vi "Process.vi"(8 "error in":errorcluster, 11 "Inst UI.Krohn-Hite-7008":refnum<class "Inst UI.Krohn-Hite-7008.lvclass">) -> (0 "error out":errorcluster, 3 "Inst UI.Krohn-Hite-7008 out":refnum<class "Inst UI.Krohn-Hite-7008.lvclass">)   [LabVIEW 2019, in "Inst UI.Krohn-Hite-7008.lvclass"]
doc: "---------------------------------------------------------------\nJKI State Machine Objects™\nhttp://jki.net/state-machine-objects/\nCopyright (C) 2005-2015, JKI <info@jki.net>\nALL RIGHTS RESERVEDJKI State Machine Objects (SMO) 1.0.0.5\nJKI - JKI\nCopyright (c) 2016, JKI"
uses:
  Inst UI.Krohn-Hite-7008.lvclass
  <vilib>/JKI/JKI SMO/SMO/SMO.lvclass
  <vilib>/JKI/JKI SMO/SMO.UI/SMO.UI.lvclass
  <userlib>/LevyLab/Instrument Framework/SMOs/Instrument/Instrument.lvclass
  Inst.Krohn-Hite-7008/Typedefs/Inst.Krohn-Hite-7008.getAll--Cluster.ctl
  Inst.Krohn-Hite-7008/Inst.Krohn-Hite-7008.lvclass
  <userlib>/LevyLab/Instrument Framework/SMOs/Instrument UI/Instrument UI.lvclass
  Inst UI.Krohn-Hite-7008.UI--Cluster.ctl
  <userlib>/LevyLab/Instrument Framework/SMOs/Configuration/Configuration.lvclass
  Inst.Krohn-Hite-7008/Typedefs/Inst.Krohn-Hite-7008.Configuration--Cluster.ctl
  <userlib>/LevyLab/Instrument Framework/SMOs/Instrument/Typedefs/Client Type--Enum.ctl
  <userlib>/LevyLab/Instrument Framework/SMOs/RemoteControl/Typedefs/Message--Cluster.ctl
  <userlib>/LevyLab/Instrument Framework/SMOs/RemoteControl/RemoteControl.lvclass
  09e9697b-516c-49fb-b2dc-692589121b6f.vi
  C:/Program Files (x86)/National Instruments/LabVIEW 2019/user.lib/LevyLab/Instrument Framework/SMOs/Instrument UI/Instrument UI.lvclass
  C:/Program Files (x86)/National Instruments/LabVIEW 2019/vi.lib/JKI/JKI SMO/SMO.UI/SMO.UI.lvclass
  C:/Program Files (x86)/National Instruments/LabVIEW 2019/vi.lib/JKI/JKI SMO/SMO/SMO.lvclass
  Inst.Krohn-Hite-7008/Typedefs/Input Configuration-Enum.ctl
  Inst.Krohn-Hite-7008/Typedefs/Coupling-Enum.ctl
  Inst.Krohn-Hite-7008/Typedefs/Shunt-Enum.ctl
  Inst.Krohn-Hite-7008/Typedefs/Filter-Enum.ctl
  Inst.Krohn-Hite-7008/Typedefs/Gain-Enum.ctl
  Inst.Krohn-Hite-7008/Typedefs/Channel-Enum.ctl
  Inst.Krohn-Hite-7008/Typedefs/SetAll-Cluster.ctl
  Inst.Krohn-Hite-7008/Typedefs/SetAll-Array.ctl
  C:/Program Files (x86)/National Instruments/LabVIEW 2019/user.lib/LevyLab/Instrument Framework/Instrument Types/VSource/Instrument.VSource.lvclass
  C:/Program Files (x86)/National Instruments/LabVIEW 2019/user.lib/LevyLab/Instrument Framework/SMOs/Instrument/Instrument.lvclass
panel:
  out "Serial No":string
  out "Model":string
  in  "Channel Setting":T1
  in  "Parameter 2":string
  out "Numeric":u32
  in  "Update":bool
  in  "Parameter":dbl
  in  "STOP":bool
  # "SMO UI Template"
  # "For instructions on how to use the JKI State Machine Objects, examples and video tutorials, visit:\nhttp://jki.net/state-machine-objects/\n\nJKI State Machine Objects™\nhttp://jki.net/state-machine-objects/\nCopyright (C) 2005-2015, JKI <info@jki.net>\nALL RIGHTS RESERVED"
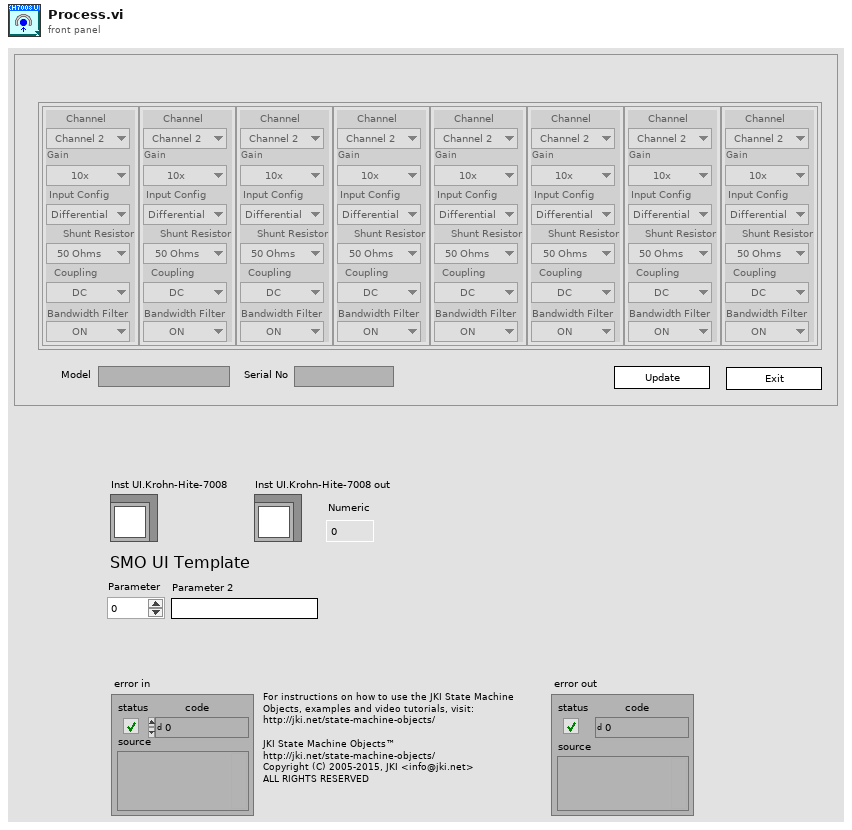
[diagram p1: front panel]
types:
  T1 = typedef "Inst.Krohn-Hite-7008.lvclass/SetAll-Array.ctl" = T2[]
  T2 = typedef "Inst.Krohn-Hite-7008.lvclass/SetAll-Cluster.ctl" = cluster{"Channel":T3, "Gain":T4, "Input Config":T5, "Shunt Resistor":T6, "Coupling":T7, "Bandwidth Filter":T8}
  T3 = typedef "Inst.Krohn-Hite-7008.lvclass/Channel-Enum.ctl" = enum16{"Channel 1", "Channel 2", "Channel 3", "Channel 4", "Channel 5", "Channel 6", "Channel 7", "Channel 8"}
  T4 = typedef "Inst.Krohn-Hite-7008.lvclass/Gain-Enum.ctl" = enum16{"1x", "10x", "100x", "1000x"}
  T5 = typedef "Inst.Krohn-Hite-7008.lvclass/Input Configuration-Enum.ctl" = enum16{"Ground", "SE+ (-gnd)", "SE- (+gnd)", "Differential"}
  T6 = typedef "Inst.Krohn-Hite-7008.lvclass/Shunt-Enum.ctl" = enum16{"Open", "50 Ohms", "500 Ohms", "5k Ohms", "50k Ohms", "10M Ohm"}
  T7 = typedef "Inst.Krohn-Hite-7008.lvclass/Coupling-Enum.ctl" = enum16{"AC", "DC"}
  T8 = typedef "Inst.Krohn-Hite-7008.lvclass/Filter-Enum.ctl" = enum16{"OFF", "ON"}
  T9 = typedef "Inst.Krohn-Hite-7008.lvclass/Inst.Krohn-Hite-7008.Configuration--Cluster.ctl" = cluster{"Visa Ref":refnum<visa-resource-name>, "Serial No":string, "Model":string}
  T10 = enum32{"invalid app kind", "Development System", "Run Time System", "Student Edition", "Embedded LabVIEW", "Evaluation", "Custom"}
  T11 = enum32{"Invalid", "Standard", "Closed", "Hidden", "Minimized", "Maximized"}
  T12 = typedef "Instrument.lvclass/Client Type--Enum.ctl" = enum16{"Remote", "Local"}
  T13 = typedef "Inst.Krohn-Hite-7008.lvclass/Inst.Krohn-Hite-7008.getAll--Cluster.ctl" = cluster{"Levy 1":dbl, "Logger SMO":dbl, "SMO Boolean":bool, "SMO String":string, "Channel Setting":T1}
  T14 = typedef "Inst UI.Krohn-Hite-7008.lvclass/Inst UI.Krohn-Hite-7008.UI--Cluster.ctl" = cluster{"Parameter":dbl, "Parameter 2":string}
  T15 = typedef "RemoteControl.lvclass/Message--Cluster.ctl" = cluster{"Command":string, "Data":variant, "ID":string}
  T16 = cluster{"Core":cluster{"Current VI Reference":refnum<vi>, "Close Panel on Exit?":bool, "Last Error":cluster{"error":errorcluster, "previous state":string, "remaining states":string}, "Shutdown?":bool}, "Instrument UI":refnum<class "Inst UI.Krohn-Hite-7008.lvclass">, "Instrument":refnum<class "Inst.Krohn-Hite-7008.lvclass">, "Configuration":refnum<class "Configuration.lvclass">, "Config Cluster":T9, "getAll":T13, "UI Cluster":T14, "Message":T15}
  T17 = cluster{"Current VI Reference":refnum<vi>, "Close Panel on Exit?":bool, "Last Error":cluster{"error":errorcluster, "previous state":string, "remaining states":string}, "Shutdown?":bool}
  T18 = typedef "SMO.lvclass/Protected Events.ctl" = cluster{"StopProcesses":refnum<user-event>, "AbortProcesses":refnum<user-event>, "Config Changed":refnum<user-event>, "Dependency":refnum<user-event>}
  T19 = typedef "Instrument.lvclass/PublicEvents--Cluster.ctl" = cluster{"MessageFromProcess":refnum<user-event>}
  T20 = typedef "Inst.Krohn-Hite-7008.lvclass/PublicEvents--Cluster.ctl" = cluster{"MessageFromProcess":refnum<user-event>}
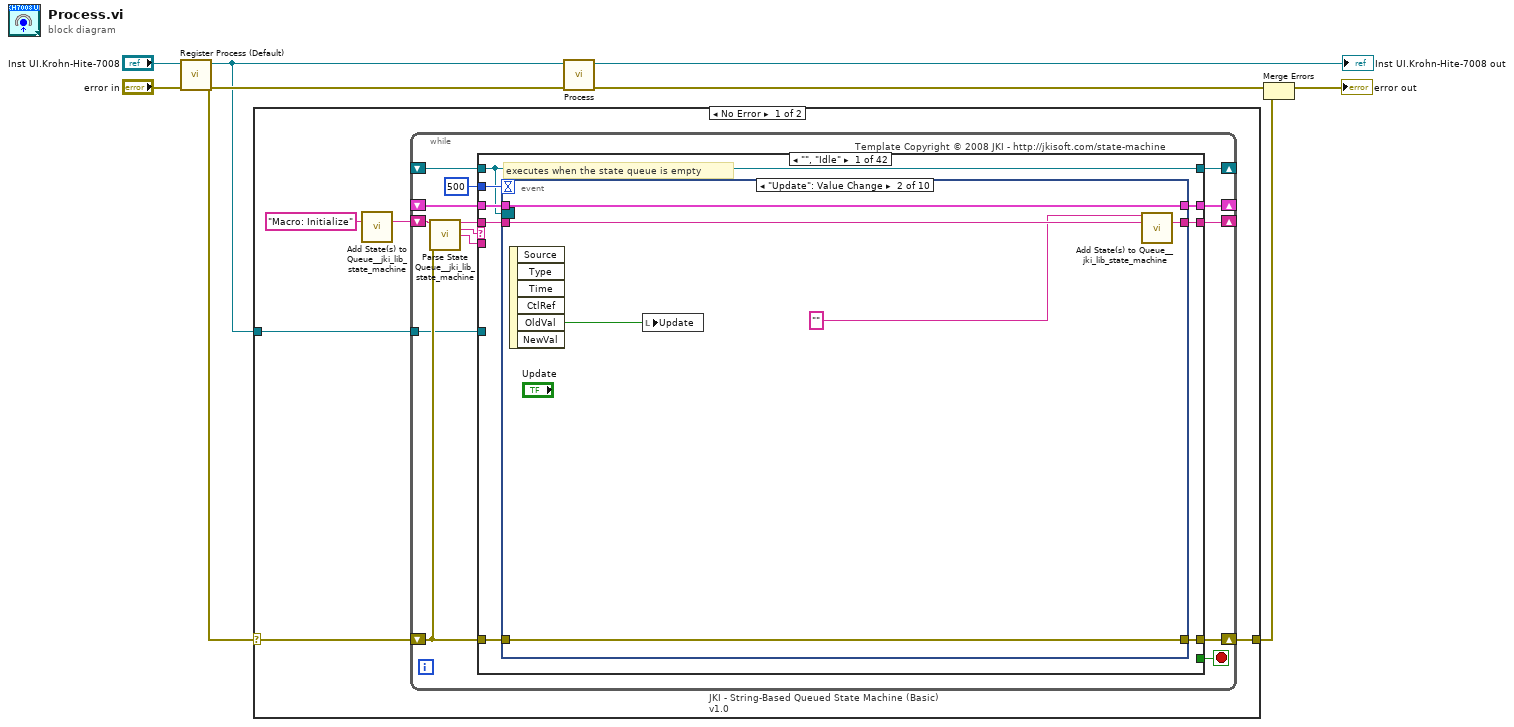
[diagram p0: block diagram]
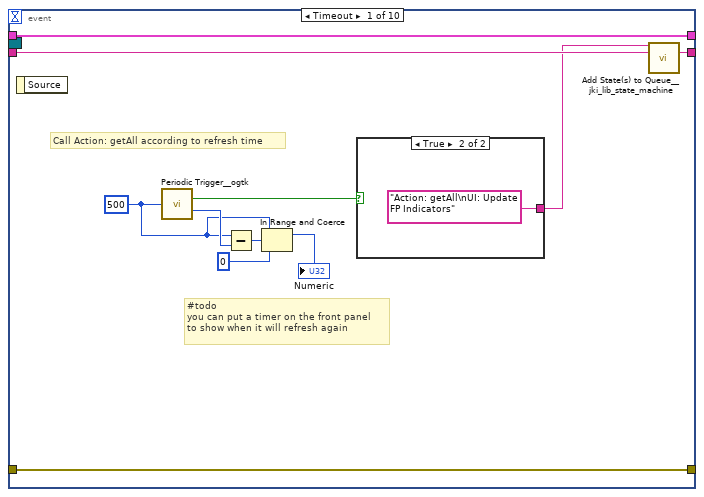
[diagram p2: hidden frame]
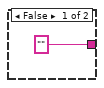
[diagram p3: hidden frame]
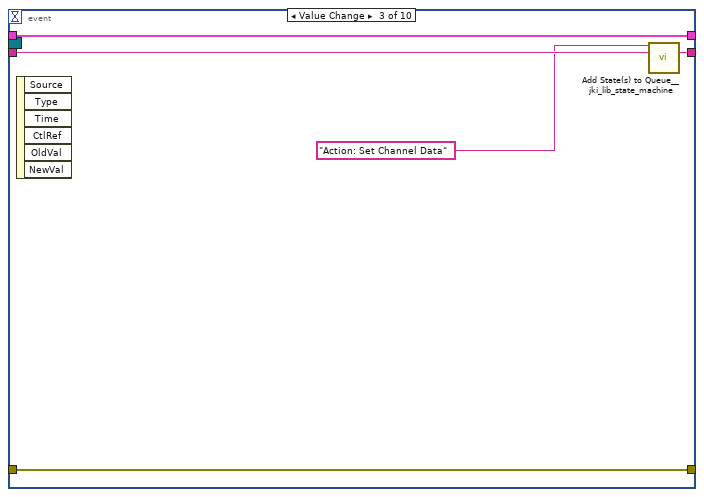
[diagram p4: hidden frame]
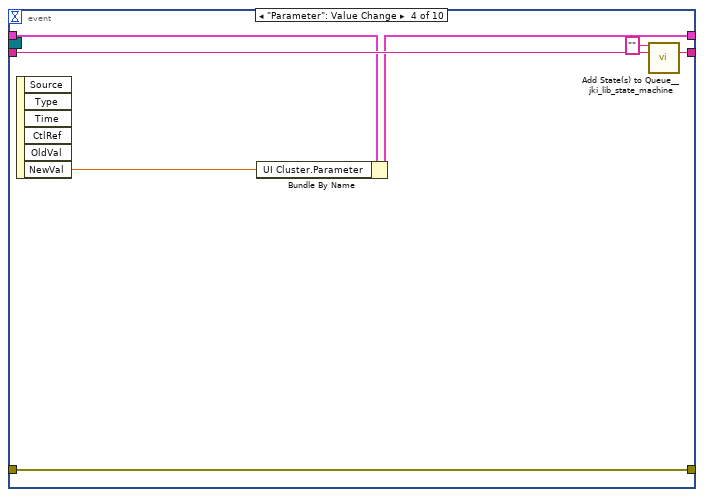
[diagram p5: hidden frame]
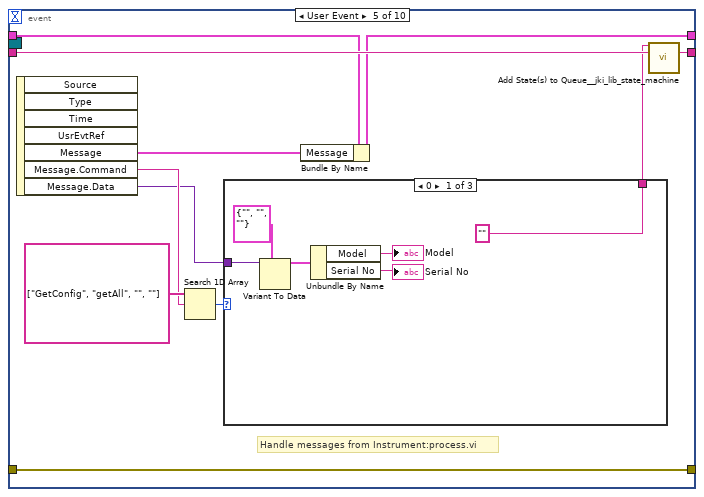
[diagram p6: hidden frame]
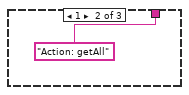
[diagram p7: hidden frame]
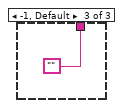
[diagram p8: hidden frame]
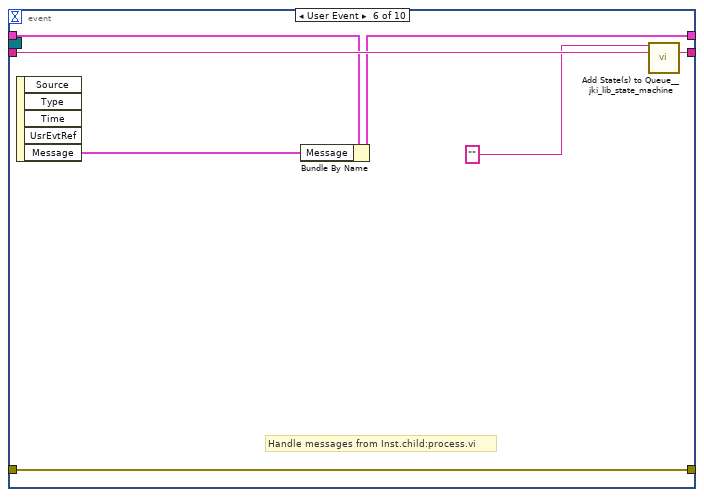
[diagram p9: hidden frame]
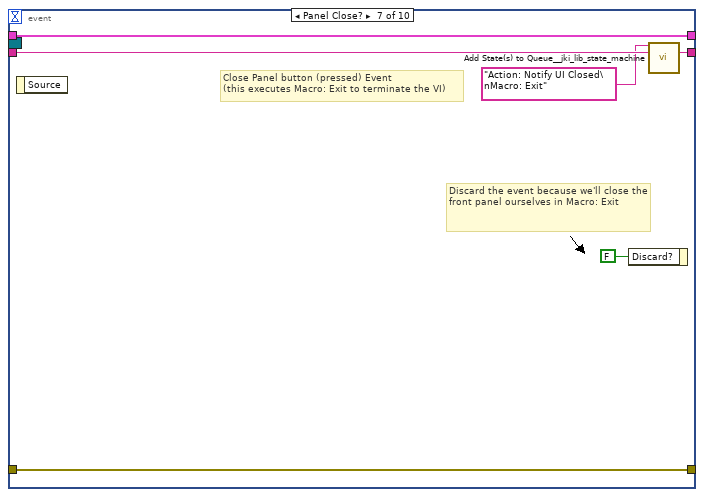
[diagram p10: hidden frame]
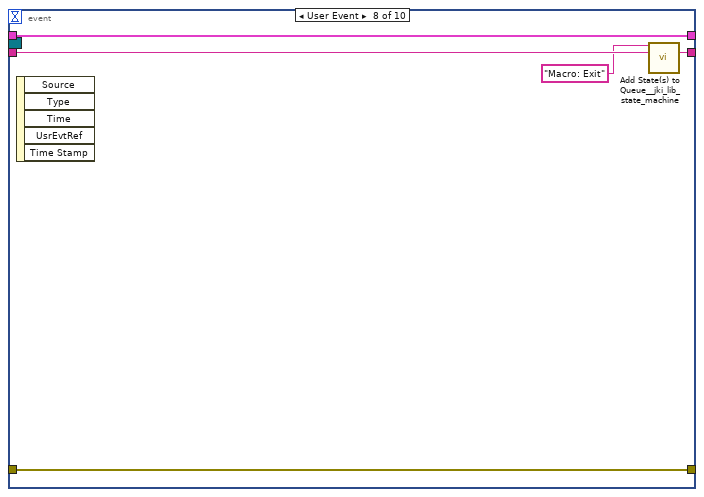
[diagram p11: hidden frame]
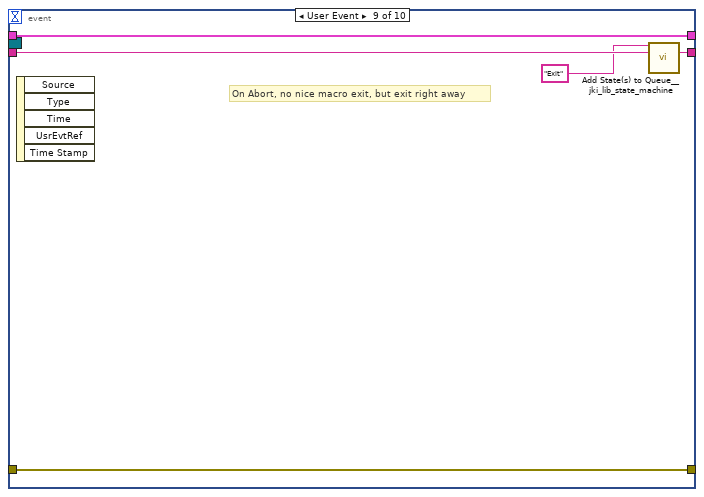
[diagram p12: hidden frame]
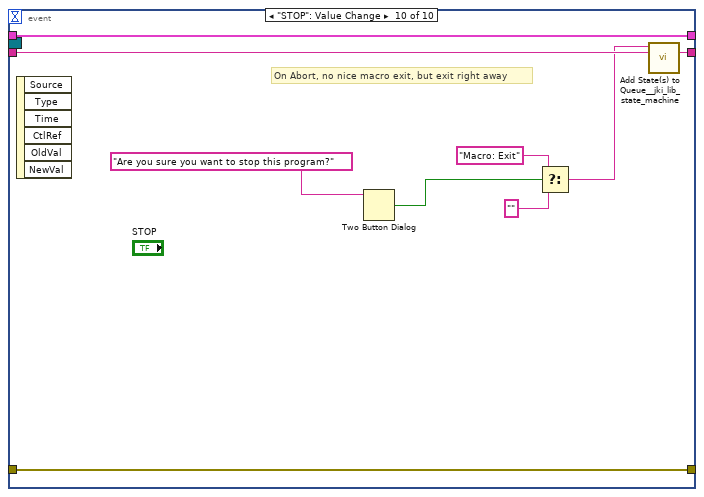
[diagram p13: hidden frame]
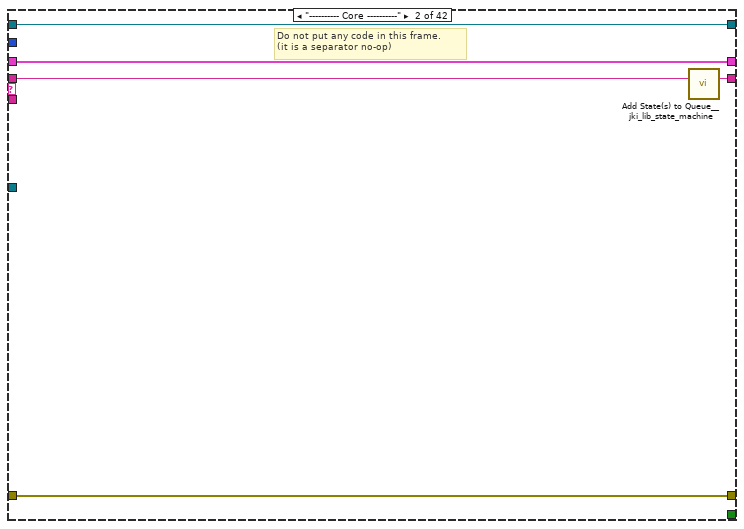
[diagram p14: hidden frame]
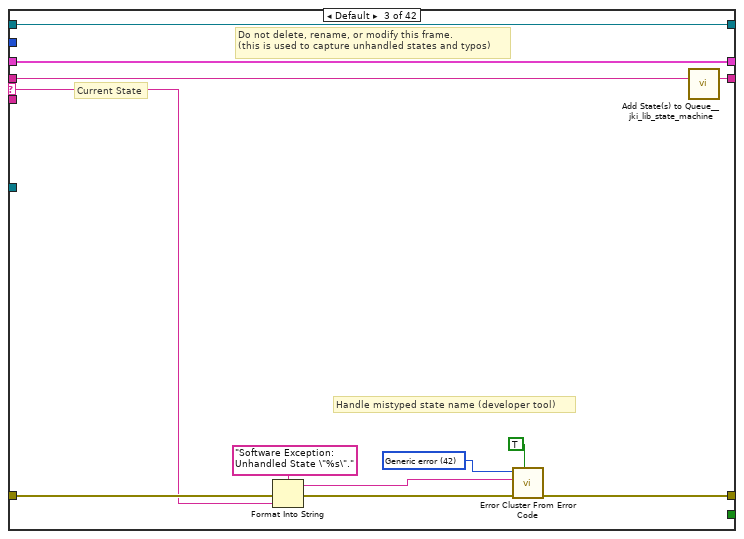
[diagram p15: hidden frame]
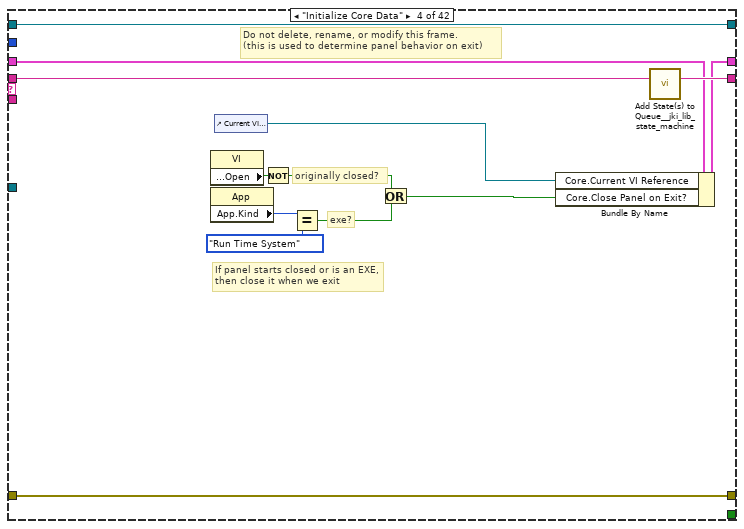
[diagram p16: hidden frame]
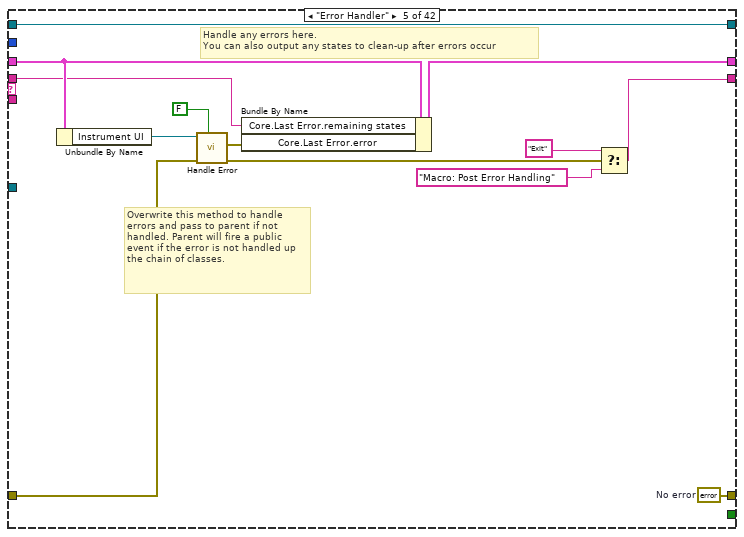
[diagram p17: hidden frame]
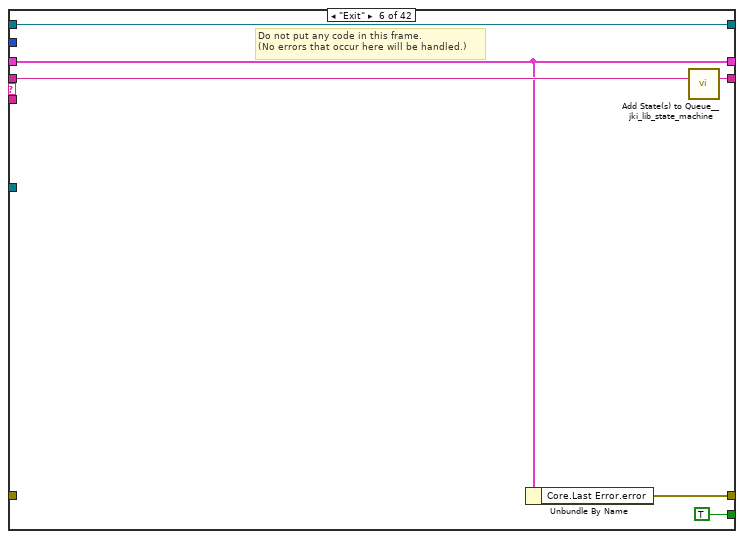
[diagram p18: hidden frame]
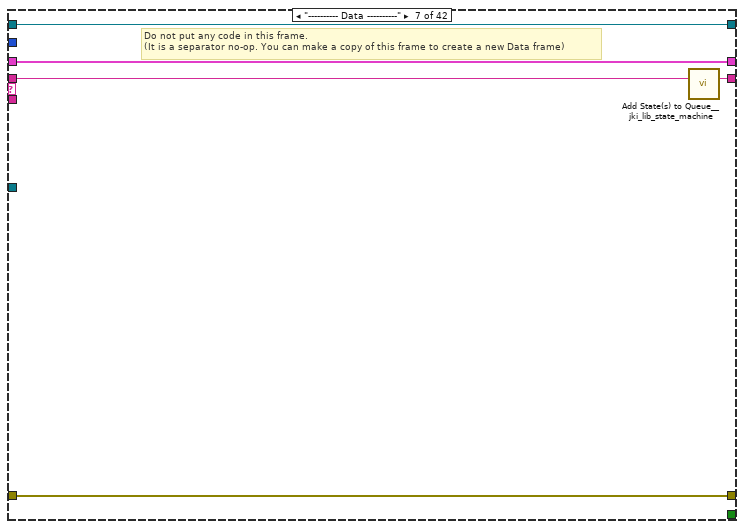
[diagram p19: hidden frame]
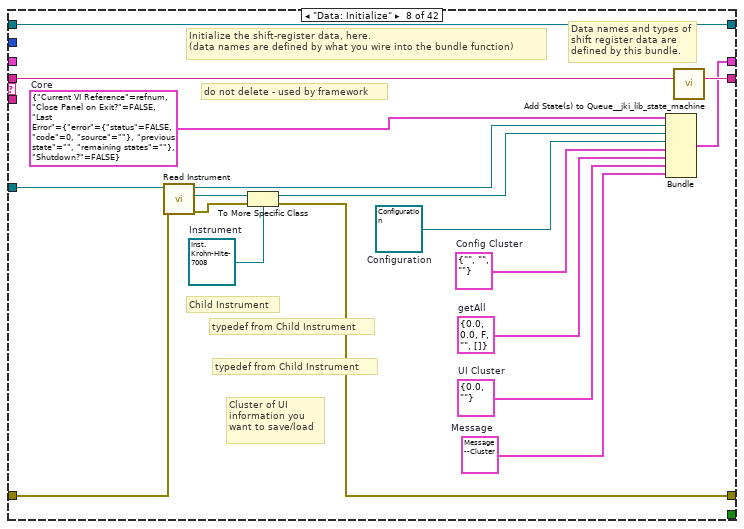
[diagram p20: hidden frame]
diagram:
  n1 = call <vilib>:"Register Process (Default).vi"("error in (no error)"="error in", "SMO"="Inst UI.Krohn-Hite-7008") -> ("error out"=w5:errorcluster, "SelfRef"=w4:refnum<class "Inst UI.Krohn-Hite-7008.lvclass">)  [unwired: 8 in]
  n2 = case shown="No Error" w5 {
    selector: w5 -> [w10 w527]
    tunnel: w4 -> [w11 _]
    tunnel: [w9 w527] -> w1
    frame No Error {
      n3 = call <vilib>:"Add State(s) to Queue__jki_lib_state_machine.vi"("State(s) in (\"\")"="Macro: Initialize") -> ("States Out"=w13:string)  [unwired: 14 in]
      n4 = while "JKI - String-Based Queued State Machine (Basic) v1.0" {
        shift-right: [w20] -> _
        shift-left: _ -> [w19]
        shift-right: [w23] -> w9
        shift-left: w10 -> [w17]
        shift-right: [w22] -> _
        shift-left: w13 -> [w24]
        tunnel: w11 -> [w16]
        shift-right: [w15] -> _
        shift-left: _ -> [w14]
        stop <- w21 stop-if-true
        # "Template Copyright © 2008 JKI - http://jkisoft.com/state-machine"
        n5 = call <vilib>:"Parse State Queue__jki_lib_state_machine.vi"("State Queue"=w24, "Error In (no error)"=w17) -> ("Remaining States"=w26:string, "Current State"=w27:string, "Arguments"=w25:string)  [unwired: 11 in]
        n6 = case shown="\"\", \"Idle\"" w27 {
          selector: w27 -> [_ _ w124 _ _ _ _ _ _ _ _ _ _ _ _ _ _ _ _ _ _ _ _ _ _ _ _ _ _ _ _ _ _ _ _ _ _ _ _ _ _ _]
          tunnel: w26 -> [w35 w122 w128 w147 w151 w166 w171 w189 w197 w204 w211 w216 w223 w230 w237 w244 w260 w292 w301 w313 w323 w329 w344 w349 w360 w367 w372 w388 w394 w399 w414 w422 w434 w441 w448 w460 w473 w483 w493 w504 w516 w526]
          tunnel: w25 -> [_ _ _ _ _ _ _ _ _ _ _ _ _ _ _ w238 w254 _ _ _ _ _ _ _ _ _ _ _ _ _ _ _ _ _ _ _ _ _ _ _ _ _]
          tunnel: w19 -> [w33 w119 w126 w138 w154 w162 w168 _ w193 w200 w205 w213 w221 w226 w232 w242 w256 w289 w297 w303 w320 w326 w331 w346 w357 w362 w369 w386 w392 w396 w407 w419 w425 w436 w442 w452 w467 w475 w488 w499 w511 w521]
          tunnel: [w32 w120 w130 w144 w156 w161 w169 w176 w195 w202 w207 w214 w218 w228 w233 w239 w257 w290 w299 w311 w321 w327 w342 w347 w351 w363 w370 w383 w389 w397 w400 w417 w426 w438 w443 w457 w470 w480 w484 w495 w507 w517] -> w23
          tunnel: w17 -> [w31 w120 w129 w144 w150 _ w169 w173 w195 w202 w208 w214 w219 w228 w233 w240 w258 w290 w299 w311 w321 w327 w342 w347 w352 w364 w370 w373 w390 w397 w409 w415 w427 w438 w444 w453 w462 w476 w485 w496 w508 w518]
          tunnel: [w34 w121 w127 w146 w148 w165 w170 w188 w196 w203 w210 w215 w222 w229 w236 w243 w259 w291 w300 w312 w322 w328 w343 w348 w359 w366 w371 w387 w393 w398 w413 w421 w433 w440 w447 w459 w472 w482 w492 w503 w515 w525] -> w22
          tunnel: [_ _ _ _ _ TRUE _ _ _ _ _ _ _ _ _ _ _ _ _ _ _ _ _ _ _ _ _ _ _ _ _ _ _ _ _ _ _ _ _ _ _ _] -> w21
          tunnel: [w30 w119 w126 w145 w153 w162 w168 w187 w192 w199 w205 w213 w221 w226 w232 w242 w256 w289 w297 w304 w320 w326 w331 w346 w357 w362 w369 w386 w392 w396 w411 w419 w423 w435 w442 w454 w468 w477 w489 w500 w512 w522] -> w20
          tunnel: 500 ("Timeout") -> [w29 _ _ _ _ _ _ _ _ _ _ _ _ _ _ _ _ _ _ _ _ _ _ _ _ _ _ _ _ _ _ _ _ _ _ _ _ _ _ _ _ _]
          tunnel: w16 -> [_ _ _ _ _ _ _ w174 _ _ _ _ _ _ _ _ _ _ _ _ _ _ _ _ _ _ _ _ _ _ _ _ _ _ _ _ _ _ _ _ _ _]
          tunnel: [w28 w118 w123 w135 w160 w163 w167 w186 w194 w201 w206 w212 w220 w227 w235 w241 w253 w288 w298 w310 w319 w325 w336 w345 w358 w365 w368 w385 w391 w395 w412 w420 w432 w439 w446 w458 w471 w481 w491 w502 w514 w524] -> w15
          tunnel: w14 -> [w28 w118 w123 w135 w160 w163 w167 w186 w194 w201 w206 w212 w220 w227 w235 w241 w253 w288 w298 w310 w319 w325 w336 w345 w358 w365 w368 _ w391 w395 w412 w420 w432 w439 w446 w458 w471 w481 w491 w502 w514 w524]
          frame "", "Idle" {
            # "executes when the state queue is empty"
            n7 = event shown="[1] \"Update\": Value Change" {
              selector: w28 -> [_ _ _ _ _ _ _ _ _ _]
              dyn-events: _ -> [_ _ _ _ _ _ _ _ _ _]
              timeout: w29 -> [_ _ _ _ _ _ _ _ _ _]
              tunnel: w35 -> [w46 w54 w59 w66 w77 w92 w98 w103 w108 w117]
              tunnel: [w45 w53 w58 w65 w76 w91 w97 w102 w107 w116] -> w34
              tunnel: w33 -> [w43 w51 w56 w62 w74 w89 w94 w100 w105 w114]
              tunnel: [w44 w52 w57 w64 w75 w90 w93 w101 w106 w115] -> w32
              tunnel: w31 -> [w44 w52 w57 w64 w75 w90 w93 w101 w106 w115]
              tunnel: [w43 w51 w56 w61 w73 w88 w94 w100 w105 w114] -> w30
              event Timeout {
                w37 = u32 500 ("time (ms)")
                # "#todo\nyou can put a timer on the front panel\nto show when it will refresh again"
                # "Call Action: getAll according to refresh time"
                n8 = event-data() -> ()  [unwired: 1 in, 1 out]
                n9 = call <userlib>:"Periodic Trigger__ogtk.vi"("time (ms)"=w37) -> ("Triggered"=w41:bool, "timer value"=w40:u32)  [unwired: 12 in, 1 out]
                n10 = Subtract(x=w37, y=w40) -> (x-y=w39:u32)
                n11 = In Range and Coerce(upper limit=w37, x=w39, lower limit=u32 0) -> (coerced(x)=→"Numeric":u32)  [unwired: 1 out]
                n12 = case shown="True" w41 {
                  tunnel: ["" ("State(s) in Front (\"\")") "Action: getAll\nUI: Update FP Indicators" ("State(s) in Front (\"\")")] -> w42
                  frame False {
                  }
                  frame True {
                  }
                }
                n13 = call <vilib>:"Add State(s) to Queue__jki_lib_state_machine.vi"("State(s) in Front (\"\")"=w42, "State(s) in (\"\")"=w46) -> ("States Out"=w45:string)  [unwired: 13 in]
              }
              event "Update": Value Change {
                n14 = event-data() -> ("OldVal"=w50:bool)  [unwired: 1 in, 5 out]
                n15 = local write "Update"(w50) -> ()
                n16 = call <vilib>:"Add State(s) to Queue__jki_lib_state_machine.vi"("State(s) in Front (\"\")"="" ("State(s) in Front (\"\")"), "State(s) in (\"\")"=w54) -> ("States Out"=w53:string)  [unwired: 13 in]
              }
              event Value Change {
                n17 = event-data() -> ()  [unwired: 1 in, 6 out]
                n18 = call <vilib>:"Add State(s) to Queue__jki_lib_state_machine.vi"("State(s) in Front (\"\")"="Action: Set Channel Data" ("State(s) in Front (\"\")"), "State(s) in (\"\")"=w59) -> ("States Out"=w58:string)  [unwired: 13 in]
              }
              event "Parameter": Value Change {
                n19 = event-data() -> ("NewVal"=w63:dbl)  [unwired: 1 in, 5 out]
                n20 = Bundle By Name(cluster=w62, "UI Cluster.Parameter"=w63) -> (w61:T16)
                n21 = call <vilib>:"Add State(s) to Queue__jki_lib_state_machine.vi"("State(s) in Front (\"\")"="" ("State(s) in Front (\"\")"), "State(s) in (\"\")"=w66) -> ("States Out"=w65:string)  [unwired: 13 in]
              }
              event User Event {
                # "Handle messages from Instrument:process.vi"
                n22 = event-data() -> ("Message"=w72:T15, "Message.Command"=w70:string, "Message.Data"=w68:variant)  [unwired: 1 in, 4 out]
                n23 = Search 1D Array(1D array=string[] ["GetConfig", "getAll", "", ""], element=w70) -> (index of element=w69:i32)  [unwired: 1 in]
                n24 = case shown="0" w69 {
                  tunnel: w68 -> [w83 _ _]
                  tunnel: ["" ("State(s) in Front (\"\")") "Action: getAll" ("State(s) in Front (\"\")") ""] -> w67
                  frame 0 {
                    n25 = Variant To Data(type=T9 {"Visa Ref"="", "Serial No"="", "Model"=""} ("Configuration"), Variant=w83) -> (data=w81:T9)  [unwired: 1 in, 1 out]
                    n26 = Unbundle By Name(w81) -> ("Model"=→"Model":string, "Serial No"=→"Serial No":string)
                  }
                  frame 1 {
                  }
                  frame -1, Default {
                  }
                }
                n27 = Bundle By Name(cluster=w74, "Message"=w72) -> (w73:T16)
                n28 = call <vilib>:"Add State(s) to Queue__jki_lib_state_machine.vi"("State(s) in Front (\"\")"=w67, "State(s) in (\"\")"=w77) -> ("States Out"=w76:string)  [unwired: 13 in]
              }
              event User Event {
                # "Handle messages from Inst.child:process.vi"
                n29 = event-data() -> ("Message"=w86:T15)  [unwired: 1 in, 4 out]
                n30 = Bundle By Name(cluster=w89, "Message"=w86) -> (w88:T16)
                n31 = call <vilib>:"Add State(s) to Queue__jki_lib_state_machine.vi"("State(s) in Front (\"\")"="" ("State(s) in Front (\"\")"), "State(s) in (\"\")"=w92) -> ("States Out"=w91:string)  [unwired: 13 in]
              }
              event Panel Close? {
                # "Discard the event because we'll close the front panel ourselves in Macro: Exit"
                # "Close Panel button (pressed) Event\n(this executes Macro: Exit to terminate the VI)"
                n32 = event-data() -> ()  [unwired: 1 in, 1 out]
                n33 = event-data("Discard?"=FALSE) -> ()  [unwired: 1 in, 1 out]
                n34 = call <vilib>:"Add State(s) to Queue__jki_lib_state_machine.vi"("State(s) in Front (\"\")"="Action: Notify UI Closed\nMacro: Exit", "State(s) in (\"\")"=w98) -> ("States Out"=w97:string)  [unwired: 13 in]
              }
              event User Event {
                n35 = event-data() -> ()  [unwired: 1 in, 5 out]
                n36 = call <vilib>:"Add State(s) to Queue__jki_lib_state_machine.vi"("State(s) in Front (\"\")"="Macro: Exit", "State(s) in (\"\")"=w103) -> ("States Out"=w102:string)  [unwired: 13 in]
              }
              event User Event {
                # "On Abort, no nice macro exit, but exit right away"
                n37 = event-data() -> ()  [unwired: 1 in, 5 out]
                n38 = call <vilib>:"Add State(s) to Queue__jki_lib_state_machine.vi"("State(s) in Front (\"\")"="Exit", "State(s) in (\"\")"=w108) -> ("States Out"=w107:string)  [unwired: 13 in]
              }
              event "STOP": Value Change {
                # "On Abort, no nice macro exit, but exit right away"
                n39 = event-data() -> ()  [unwired: 1 in, 6 out]
                n40 = Two Button Dialog(message="Are you sure you want to stop this program?") -> (T button?=w113:bool)  [unwired: 2 in]
                n41 = Select(t="Macro: Exit", s=w113, f="") -> (s? t:f=w109:string)
                n42 = call <vilib>:"Add State(s) to Queue__jki_lib_state_machine.vi"("State(s) in Front (\"\")"=w109, "State(s) in (\"\")"=w117) -> ("States Out"=w116:string)  [unwired: 13 in]
              }
            }
          }
          frame "---------- Core ----------" {
            # "Do not put any code in this frame.\n(it is a separator no-op)"
            n43 = call <vilib>:"Add State(s) to Queue__jki_lib_state_machine.vi"("State(s) in (\"\")"=w122) -> ("States Out"=w121:string)  [unwired: 14 in]
          }
          frame Default {
            w133 = 42 items=["No error", "Argument error", "Memory is full", "Out of zone", "End of file", "File already open", "Generic file I/O error", "File not found", "File permission error", "Disk is full", "Duplicate path", "Too many files open", "System feature not enabled", "Resource file not found", "Cannot add resource", "Resource not found", "Image not found", "Image memory error", "Pen does not exist", "Config type invalid", "Config token not found", "Config parse error", "Config memory error", "Bad external code format", "Bad external code offset", "External code not present", "Null window", "Destroy window error", "Null menu", "Print aborted", "Bad print record", "Print driver error", "Windows error during printing", "Memory error during printing", "Print dialog error", "Generic print error", "Invalid device refnum", "Device not found", "Device parameter error", "Device unit error", "Cannot open device", "Device call aborted", "Generic error", "Cancelled by user", "Object ID too low", "Object ID too high", "Object not in heap", "Unknown heap", "Unknown object (invalid DefProc)", "Unknown object (DefProc not in table)", "Message out of range", "Invalid (null) method", "Unknown message", "Manager call not supported", "Bad address", "Network operation in progress", "Network operation timed out", "Connection is busy", "Network attribute not supported", "Network error", "Address in use", "System out of memory", "Connection aborted", "Connection refused", "Not connected", "Already connected", "Connection closed", "Initialization error (interapplication manager)", "Bad occurrence", "Wait on unbound occurrence handler", "Occurrence queue overflow", "Datalog type conflict", "Unused", "Unrecognized type (interapplication manager)", "Memory corrupt", "Failed to make temporary DLL", "Old CIN version", "Drag socket not found", "Failed to load drop-object", "Failed to register OLE object", "Failed to release OLE object", "Format specifier type mismatch", "Unknown format specifier", "Too few format specifiers", "Too many format specifiers", "Scan failed", "Newer CIN version", "Error converting to variant", "Runtime menu error", "Password tampered", "Variant attribute not found", "Incompatible variant data type", "Event data is not available", "Event Store is not present", "Occurrence is not found", "Event Queue is not created", "Event info is not available", "Refnum passed is NULL", "Error retrieving Class GUID", "Error retrieving CoClass GUID", "Error retrieving TypeLib GUID.", "Bad built application magic bytes.", "Specific driver is different from the specific driver associated with the Logical Name.", "There is no session opened to the class driver.", "Max Error", "MAX - Error with config objects", "MAX - Error loading configuration", "MAX - Group not supported"]
            # "Current State"
            # "Do not delete, rename, or modify this frame.\n(this is used to capture unhandled states and typos)"
            # "Handle mistyped state name (developer tool)"
            n44 = Format Into String(format string="Software Exception: Unhandled State \"%s\"." ("message"), error in=w129, w124) -> (resulting string=w132:string, error out=w131:errorcluster)  [unwired: 1 in]
            n45 = call <vilib>:"Error Cluster From Error Code.vi"("show call chain? (False)"=TRUE, "error in (no error)"=w131, "error message (\"\")"=w132, "error code (0)"=w133) -> ("error out"=w130:errorcluster)  [unwired: 5 in]
            n46 = call <vilib>:"Add State(s) to Queue__jki_lib_state_machine.vi"("State(s) in (\"\")"=w128) -> ("States Out"=w127:string)  [unwired: 14 in]
          }
          frame "Initialize Core Data" {
            # "Do not delete, rename, or modify this frame.\n(this is used to determine panel behavior on exit)"
            # "originally closed?"
            # "exe?"
            # "If panel starts closed or is an EXE, then close it when we exit"
            n47 = property class="VI"() -> ("Front Panel.Open"=w143:bool)  [unwired: 2 in, 2 out]
            n48 = property class="App"() -> ("App.Kind"=w142:T10)  [unwired: 2 in, 2 out]
            n49 = control-ref of="Current VI Reference"() -> (w136:refnum<vi>)
            n50 = Not(x=w143) -> (.not. x?=w140:bool)
            n51 = Equal?(x=w142, y=T10."Run Time System" ("Application:Kind")) -> (x = y?=w139:bool)
            n52 = Or(x=w140, y=w139) -> (x .or. y?=w137:bool)
            n53 = Bundle By Name(cluster=w138, "Core.Current VI Reference"=w136, "Core.Close Panel on Exit?"=w137) -> (w145:T16)
            n54 = call <vilib>:"Add State(s) to Queue__jki_lib_state_machine.vi"("State(s) in (\"\")"=w147) -> ("States Out"=w146:string)  [unwired: 14 in]
          }
          frame "Error Handler" {
            w156 = errorcluster {"status"=FALSE, "code"=0, "source"=""}  # No error
            # "Overwrite this method to handle errors and pass to parent if not handled. Parent will fire a public event if the error is not handled up the chain of classes."
            # "Handle any errors here.\nYou can also output any states to clean-up after errors occur"
            n55 = Unbundle By Name(w154) -> ("Instrument UI"=w159:refnum<class "Inst UI.Krohn-Hite-7008.lvclass">)
            n56 = call-dynamic "Handle Error.vi"("Stop on Unhandled Error (T)"=FALSE, "error in"=w150, "SMO"=w159) -> ("handling error"=w157:errorcluster, "Unhandled error"=w155:errorcluster)  [unwired: 6 in, 1 out]
            n57 = Bundle By Name(cluster=w154, "Core.Last Error.remaining states"=w151, "Core.Last Error.error"=w155) -> (w153:T16)
            n58 = Select(t="Exit", s=w157, f="Macro: Post Error Handling") -> (s? t:f=w148:string)
          }
          frame "Exit" {
            # "Do not put any code in this frame.\n(No errors that occur here will be handled.)"
            n59 = Unbundle By Name(w162) -> ("Core.Last Error.error"=w161:errorcluster)
            n60 = call <vilib>:"Add State(s) to Queue__jki_lib_state_machine.vi"("State(s) in (\"\")"=w166) -> ("States Out"=w165:string)  [unwired: 14 in]
          }
          frame "---------- Data ----------" {
            # "Do not put any code in this frame.\n(It is a separator no-op. You can make a copy of this frame to create a new Data frame)"
            n61 = call <vilib>:"Add State(s) to Queue__jki_lib_state_machine.vi"("State(s) in (\"\")"=w171) -> ("States Out"=w170:string)  [unwired: 14 in]
          }
          frame "Data: Initialize" {
            w172 = T15 {"Command"="", "Data"=variant, "ID"=""}  # Message
            w175 = refnum<class "Configuration.lvclass"> refnum  # Configuration
            w178 = T9 {"Visa Ref"="", "Serial No"="", "Model"=""}  # Config Cluster
            w180 = T14 {"Parameter"=0.0, "Parameter 2"=""}  # UI Cluster
            w182 = refnum<class "Inst.Krohn-Hite-7008.lvclass"> refnum  # Instrument
            w184 = T13 {"Levy 1"=0.0, "Logger SMO"=0.0, "SMO Boolean"=FALSE, "SMO String"="", "Channel Setting"=[]}  # getAll
            w185 = T17 {"Current VI Reference"=refnum, "Close Panel on Exit?"=FALSE, "Last Error"={"error"={"status"=FALSE, "code"=0, "source"=""}, "previous state"="", "remaining states"=""}, "Shutdown?"=FALSE}  # Core
            # "typedef from Child Instrument"
            # "Cluster of UI\ninformation you\nwant to save/load"
            # "Child Instrument"
            # "typedef from Child Instrument"
            # "do not delete - used by framework"
            # "Data names and types of shift register data are defined by this bundle."
            # "Initialize the shift-register data, here.\n(data names are defined by what you wire into the bundle function)"
            n62 = call <userlib>:"Read Instrument.vi"("error in (no error)"=w173, "Instrument UI in"=w174) -> ("error out"=w179:errorcluster, "Instrument"=w181:refnum<class "Instrument.lvclass">, "Instrument UI"=w183:refnum<class "Inst UI.Krohn-Hite-7008.lvclass">)  [unwired: 7 in]
            n63 = To More Specific Class(target class=w182, reference=w181, error in=w179) -> (specific class reference=w177:refnum<class "Inst.Krohn-Hite-7008.lvclass">, error out=w176:errorcluster)
            n64 = Bundle("Core"=w185, "Instrument UI"=w183, "Instrument"=w177, "Configuration"=w175, "Config Cluster"=w178, "getAll"=w184, "UI Cluster"=w180, "Message"=w172) -> (w187:T16)  [unwired: 1 in]
            n65 = call <vilib>:"Add State(s) to Queue__jki_lib_state_machine.vi"("State(s) in (\"\")"=w189) -> ("States Out"=w188:string)  [unwired: 14 in]
          }
          frame "Data: Set UI Cluster" {
            # "Do not put any code in this frame.\n(It is a separator no-op. You can make a copy of this frame to create a new Data frame)"
            n66 = Bundle By Name(cluster=w193, "UI Cluster.Parameter"="Parameter", "UI Cluster.Parameter 2"="Parameter 2") -> (w192:T16)
            n67 = call <vilib>:"Add State(s) to Queue__jki_lib_state_machine.vi"("State(s) in (\"\")"=w197) -> ("States Out"=w196:string)  [unwired: 14 in]
          }
          frame "Data: Set Config Cluster" {
            # "Do not put any code in this frame.\n(It is a separator no-op. You can make a copy of this frame to create a new Data frame)"
            n68 = Unbundle By Name(w200) -> ("Config Cluster"=w198:T9)
            n69 = Bundle By Name(cluster=w200, "Config Cluster"=w198) -> (w199:T16)
            n70 = call <vilib>:"Add State(s) to Queue__jki_lib_state_machine.vi"("State(s) in (\"\")"=w204) -> ("States Out"=w203:string)  [unwired: 14 in]
          }
          frame "Data: Cleanup" {
            # "Cleanup any data and references, here.\n(this is called automatically, by the Macro: Exit)"
            n71 = Unbundle By Name(w205) -> ("Core.Current VI Reference"=w209:refnum<vi>)
            n72 = Close Reference(reference=w209, error in (no error)=w208) -> (error out=w207:errorcluster)
            n73 = call <vilib>:"Add State(s) to Queue__jki_lib_state_machine.vi"("State(s) in (\"\")"=w211) -> ("States Out"=w210:string)  [unwired: 14 in]
          }
          frame "---------- UI ----------" {
            # "Do not put any code in this frame.\n(It is a separator no-op. You can make a copy of this frame to create a new UI frame)"
            n74 = call <vilib>:"Add State(s) to Queue__jki_lib_state_machine.vi"("State(s) in (\"\")"=w216) -> ("States Out"=w215:string)  [unwired: 14 in]
          }
          frame "UI: Initialize" {
            # "size window to decoration box on front panel"
            # "Initialize the User Interface, here.\n(this is called automatically, by the Macro: Init)"
            n75 = invoke on="STOP" class="Bool (strict)" method="Reinit To Default"() -> ()  [unwired: 3 in, 3 out]
            n76 = call <userlib>:"Fit VI window to Largest Dec__ogtk.vi"("error in (no error)"=w219, "border spacing (2 px)"=0) -> ("error out"=w218:errorcluster)  [unwired: 4 in, 1 out]
            n77 = call <vilib>:"Add State(s) to Queue__jki_lib_state_machine.vi"("State(s) in (\"\")"=w223) -> ("States Out"=w222:string)  [unwired: 14 in]
          }
          frame "UI: Update FP Controls" {
            # "Do not put any code in this frame.\n(It is a separator no-op. You can make a copy of this frame to create a new UI frame)"
            n78 = Unbundle By Name(w226) -> ("UI Cluster.Parameter"=w224:dbl, "UI Cluster.Parameter 2"=w225:string)
            n79 = local write "Parameter 2"(w225) -> ()
            n80 = local write "Parameter"(w224) -> ()
            n81 = call <vilib>:"Add State(s) to Queue__jki_lib_state_machine.vi"("State(s) in (\"\")"=w230) -> ("States Out"=w229:string)  [unwired: 14 in]
          }
          frame "UI: Update FP Indicators" {
            n82 = Unbundle By Name(w232) -> ("getAll"=w234:T13)
            n83 = Unbundle By Name(w234) -> ("Channel Setting"=w231:T1)
            n84 = local write "Channel Setting"(w231) -> ()
            n85 = call <vilib>:"Add State(s) to Queue__jki_lib_state_machine.vi"("State(s) in (\"\")"=w237) -> ("States Out"=w236:string)  [unwired: 14 in]
          }
          frame "UI: Cursor Set" {
            # "Argument"
            # "Initialize the User Interface, here.\n(this is called automatically, by the Macro: Init)"
            n86 = disable-structure shown="Default" {
              disable-tunnel: w240 -> [w245 w248]
              disable-tunnel: [w245 w247] -> w239
              disable-tunnel: w238 -> [_ w246]
              frame condition #0 {
              }
              frame condition #1 (active) {
                n87 = case shown="\"Busy\"" w246 {
                  tunnel: w248 -> [w250 w252]
                  tunnel: [w249 w251] -> w247
                  frame "Idle", Default {
                    n88 = call <vilib>:"Unset Busy.vi"("error in (no error)"=w250) -> ("error out"=w249:errorcluster)  [unwired: 10 in]
                  }
                  frame "Busy" {
                    n89 = call <vilib>:"Set Busy.vi"("error in (no error)"=w252) -> ("error out"=w251:errorcluster)  [unwired: 9 in, 1 out]
                  }
                }
              }
            }
            n90 = call <vilib>:"Add State(s) to Queue__jki_lib_state_machine.vi"("State(s) in (\"\")"=w244) -> ("States Out"=w243:string)  [unwired: 14 in]
          }
          frame "UI: Front Panel State" {
            # "Argument"
            # "Set Front Panel Open or Closed\n(Usage: \"UI: Front Panel State >> Open|Close\")"
            n91 = Unbundle By Name(w256) -> ("Core.Current VI Reference"=w255:refnum<vi>)
            n92 = disable-structure shown="Default" {
              disable-tunnel: w258 -> [w264 w287]
              disable-tunnel: [w263 w287] -> w257
              disable-tunnel: w255 -> [w262 _]
              disable-tunnel: w254 -> [w261 _]
              frame condition #0 (active) {
                n93 = case shown="\"Close\"" w261 {
                  tunnel: w264 -> [w268 w281]
                  tunnel: [w270 w282] -> w263
                  tunnel: w262 -> [w269 w279]
                  frame "Open", Default {
                    n94 = property class="VI"(reference=w269, error in=w268) -> (reference out=w266:refnum<vi>, error out=w267:errorcluster, "FP.State"=w265:T11)
                    n95 = case shown="\"Closed\"" w265 {
                      tunnel: [w273 w276] -> w270
                      tunnel: w267 -> [w272 w276]
                      tunnel: w266 -> [w271 _]
                      frame "Closed" {
                        n96 = invoke class="VI" method="FP.Open"(reference=w271, error in=w272, "Activate"=TRUE, "State"=T11."Standard") -> (error out=w273:errorcluster)  [unwired: 1 in, 4 out]
                      }
                      frame Default {
                      }
                    }
                  }
                  frame "Close" {
                    n97 = property class="VI"(reference=w279, error in=w281) -> (reference out=w278:refnum<vi>, error out=w280:errorcluster, "FP.State"=w277:T11)
                    n98 = case shown="Default" w277 {
                      tunnel: [w283 w286] -> w282
                      tunnel: w280 -> [w283 w285]
                      tunnel: w278 -> [_ w284]
                      frame "Invalid", "Closed" {
                      }
                      frame Default {
                        n99 = invoke class="VI" method="FP.Close"(reference=w284, error in=w285) -> (error out=w286:errorcluster)  [unwired: 1 in, 2 out]
                      }
                    }
                  }
                }
              }
              frame condition #1 {
              }
            }
            n100 = call <vilib>:"Add State(s) to Queue__jki_lib_state_machine.vi"("State(s) in (\"\")"=w260) -> ("States Out"=w259:string)  [unwired: 14 in]
          }
          frame "---------- Macro ----------" {
            # "Do not put any code in this frame.\n(It is a separator no-op. You can make a copy of this frame to create a new Macro frame)"
            n101 = call <vilib>:"Add State(s) to Queue__jki_lib_state_machine.vi"("State(s) in (\"\")"=w292) -> ("States Out"=w291:string)  [unwired: 14 in]
          }
          frame "Macro: Initialize" {
            w295 = "UI: Initialize\nMacro: Read UI Config\nAction: Open\nAction: GetConfig\n//UI: Front Panel State >> Open"  # UI: Initialize Macro: Read UI Config Action: Open Action: GetConfig //UI: Front Panel State >> Open
            # "Initialization Macro\n(This is called once, when the VI starts)"
            n102 = call <vilib>:"Add State(s) to Queue__jki_lib_state_machine.vi"("State(s) in Front (\"\")"="Data: Initialize\nInitialize Core Data\nEvents: Register", "State(s) in (\"\")"="Process: Sync", "State(s) at Back (\"\")"=w295) -> ("States Out"=w294:string)  [unwired: 12 in]
            n103 = call <vilib>:"Add State(s) to Queue__jki_lib_state_machine.vi"("State(s) in Front (\"\")"=w294, "State(s) in (\"\")"=w301) -> ("States Out"=w300:string)  [unwired: 13 in]
          }
          frame "Macro: Post Error Handling" {
            # "Clear Last Error?"
            n104 = Unbundle By Name(w303) -> ("Core.Last Error.remaining states"=w305:string, "Core.Shutdown?"=w306:bool)
            n105 = Unbundle By Name(w303) -> ("Core.Last Error.error"=w309:errorcluster)
            n106 = case shown="False" FALSE {
              tunnel: w309 -> [w317 _]
              tunnel: [w317 _] -> w308
              frame False {
              }
              frame True {
              }
            }
            n107 = case shown="True" w306 {
              tunnel: w305 -> [w314 w316]
              tunnel: [w314 w315] -> w302
              frame False {
                # "These are the remaining states (at the moment the error occured). States can be altered according to business logic."
                # "NOT SHUTTING DOWN"
              }
              frame True {
                # "Developer can decide to alter the states but should be aware that during the shutdown process, there are certain states that must be run for the SMO to properly shut itself (and this process) down. As such, one can add states to perform additional clean-ups, but should append the remaining state to be executed."
                # "SHUTTING DOWN"
                n108 = call <vilib>:"Add State(s) to Queue__jki_lib_state_machine.vi"("State(s) in (\"\")"=w316) -> ("States Out"=w315:string)  [unwired: 14 in]
              }
            }
            n109 = Bundle By Name(cluster=w303, "Core.Last Error.error"=w308) -> (w304:T16)
            n110 = call <vilib>:"Add State(s) to Queue__jki_lib_state_machine.vi"("State(s) in Front (\"\")"=w302, "State(s) in (\"\")"=w313) -> ("States Out"=w312:string)  [unwired: 13 in]
          }
          frame "Macro: Read UI Config" {
            # "Do not put any code in this frame.\n(It is a separator no-op. You can make a copy of this frame to create a new Macro frame)"
            n111 = call <vilib>:"Add State(s) to Queue__jki_lib_state_machine.vi"("State(s) in Front (\"\")"="Configuration: Initialize\nConfiguration: Read UI Config File\nUI: Update FP Controls" ("State(s) in Front (\"\")"), "State(s) in (\"\")"=w323) -> ("States Out"=w322:string)  [unwired: 13 in]
          }
          frame "Macro: Write UI Config" {
            # "Do not put any code in this frame.\n(It is a separator no-op. You can make a copy of this frame to create a new Macro frame)"
            n112 = call <vilib>:"Add State(s) to Queue__jki_lib_state_machine.vi"("State(s) in Front (\"\")"="Data: Set UI Cluster\nConfiguration: Write UI Config File" ("State(s) in Front (\"\")"), "State(s) in (\"\")"=w329) -> ("States Out"=w328:string)  [unwired: 13 in]
          }
          frame "Macro: Exit" {
            # "Exit Macro\n(This is called once, when the VI exits)"
            n113 = Unbundle By Name(w331) -> ("Core.Close Panel on Exit?"=w341:bool)
            n114 = Select(t="UI: Front Panel State >> Close", s=w341, f="" ("Empty String Constant")) -> (s? t:f=w338:string)
            n115 = call <vilib>:"Add State(s) to Queue__jki_lib_state_machine.vi"("State(s) in Front (\"\")"="Data: Cleanup\nEvents: Unregister\nProcess: Self Terminate", "State(s) in (\"\")"="Process: Sync", "State(s) at Back (\"\")"="Exit") -> ("States Out"=w333:string)  [unwired: 12 in]
            n116 = call <vilib>:"Add State(s) to Queue__jki_lib_state_machine.vi"("State(s) in Front (\"\")"="Action: Close\nMacro: Write UI Config", "State(s) in (\"\")"=w338, "State(s) at Back (\"\")"=w333) -> ("States Out"=w337:string)  [unwired: 12 in]
            n117 = call <vilib>:"Add State(s) to Queue__jki_lib_state_machine.vi"("State(s) in Front (\"\")"=w337, "State(s) in (\"\")"=w344) -> ("States Out"=w343:string)  [unwired: 13 in]
          }
          frame "---------- Process ----------" {
            # "Template Separator\n(You can make a copy of, or modify, this frame)"
            n118 = call <vilib>:"Add State(s) to Queue__jki_lib_state_machine.vi"("State(s) in (\"\")"=w349) -> ("States Out"=w348:string)  [unwired: 14 in]
          }
          frame "Process: Sync" {
            n119 = Unbundle By Name(w357) -> ("Instrument UI"=w353:refnum<class "Inst UI.Krohn-Hite-7008.lvclass">)
            n120 = call <vilib>:"WaitOnProcessSync.vi"("error in (no error)"=w352, "SMO"=w353) -> ("error out"=w351:errorcluster, "Don't run?"=w356:bool)  [unwired: 7 in, 1 out]
            n121 = Select(t="Data: Cleanup\nEvents: Unregister\nExit", s=w356, f="" ("Empty String Constant")) -> (s? t:f=w350:string)
            n122 = call <vilib>:"Add State(s) to Queue__jki_lib_state_machine.vi"("State(s) in Front (\"\")"=w350, "State(s) in (\"\")"=w360) -> ("States Out"=w359:string)  [unwired: 13 in]
          }
          frame "Process: Self Terminate" {
            n123 = Unbundle By Name(w362) -> ("Instrument UI"=w361:refnum<class "Inst UI.Krohn-Hite-7008.lvclass">)
            n124 = call <vilib>:"SelfTerminate.vi"("error in (no error)"=w364, "SMO in"=w361) -> ("error out"=w363:errorcluster)  [unwired: 8 in, 1 out]
            n125 = call <vilib>:"Add State(s) to Queue__jki_lib_state_machine.vi"("State(s) in (\"\")"=w367) -> ("States Out"=w366:string)  [unwired: 14 in]
          }
          frame "---------- Events ----------" {
            # "Template Separator\n(You can make a copy of, or modify, this frame)"
            n126 = call <vilib>:"Add State(s) to Queue__jki_lib_state_machine.vi"("State(s) in (\"\")"=w372) -> ("States Out"=w371:string)  [unwired: 14 in]
          }
          frame "Events: Register" {
            # "Expand to add\nmore events"
            # "Base Class Protected Events"
            n127 = Unbundle By Name(w386) -> ("Instrument UI"=w379:refnum<class "Inst UI.Krohn-Hite-7008.lvclass">, "Instrument"=w378:refnum<class "Inst.Krohn-Hite-7008.lvclass">)
            n128 = call <vilib>:"GetProtectedEvents.vi"("SMO"=w379) -> ("error out"=w382:errorcluster, "SMO Protected Events"=w384:T18)  [unwired: 8 in, 1 out]
            n129 = call <userlib>:"Instrument.GetPublicEvents.vi"("Instrument"=w378) -> ("error out"=w380:errorcluster, "Instrument Public Events"=w381:T19, "Instrument out"=w376:refnum<class "Inst.Krohn-Hite-7008.lvclass">)  [unwired: 8 in]
            n130 = call "Inst.Krohn-Hite-7008.GetPublicEvents.vi"("Inst.Krohn-Hite-7008 in"=w376) -> ("error out"=w375:errorcluster, "Inst.Krohn-Hite-7008 Public Events"=w377:T20)  [unwired: 8 in, 1 out]
            n131 = register-events(w384, w381, w377) -> (reference out=w385:refnum<event-registration>, error out=w374:errorcluster)  [unwired: 2 in]
            n132 = Merge Errors(w374, w375, w380, w382, w373) -> (w383:errorcluster)
            n133 = call <vilib>:"Add State(s) to Queue__jki_lib_state_machine.vi"("State(s) in (\"\")"=w388) -> ("States Out"=w387:string)  [unwired: 14 in]
          }
          frame "Events: Unregister" {
            n134 = Unregister For Events(event registration refnum=w391, error in=w390) -> (error out=w389:errorcluster)
            n135 = call <vilib>:"Add State(s) to Queue__jki_lib_state_machine.vi"("State(s) in (\"\")"=w394) -> ("States Out"=w393:string)  [unwired: 14 in]
          }
          frame "---------- Configuration ----------" {
            # "Do not put any code in this frame.\n(It is a separator no-op. You can make a copy of this frame to create a new UI frame)"
            n136 = call <vilib>:"Add State(s) to Queue__jki_lib_state_machine.vi"("State(s) in (\"\")"=w399) -> ("States Out"=w398:string)  [unwired: 14 in]
          }
          frame "Configuration: Initialize" {
            # "Do not put any code in this frame.\n(It is a separator no-op. You can make a copy of this frame to create a new UI frame)"
            n137 = Unbundle By Name(w407) -> ("Configuration"=w405:refnum<class "Configuration.lvclass">, "Instrument"=w406:refnum<class "Inst.Krohn-Hite-7008.lvclass">)
            n138 = call <vilib>:"GetName.vi"("error in (no error)"=w409, "SMO"=w406) -> ("error out"=w408:errorcluster, "Name"=w410:string)  [unwired: 6 in, 2 out]
            n139 = call <userlib>:"Default Path.vi"("error in (no error)"=w408, "Folder Name [Application Name]"=w410, "Configuration in"=w405) -> ("error out"=w401:errorcluster, "Configuration out"=w404:refnum<class "Configuration.lvclass">)  [unwired: 7 in]
            n140 = call <userlib>:"Write Section.vi"("error in (no error)"=w401, "Section"="UI", "Configuration in"=w404) -> ("error out"=w400:errorcluster, "Configuration out"=w403:refnum<class "Configuration.lvclass">)  [unwired: 7 in]
            n141 = Bundle By Name(cluster=w407, "Configuration"=w403) -> (w411:T16)
            n142 = call <vilib>:"Add State(s) to Queue__jki_lib_state_machine.vi"("State(s) in (\"\")"=w414) -> ("States Out"=w413:string)  [unwired: 14 in]
          }
          frame "Configuration: Write UI Config File" {
            # "Do not put any code in this frame.\n(It is a separator no-op. You can make a copy of this frame to create a new Data frame)"
            n143 = Unbundle By Name(w419) -> ("Configuration"=w416:refnum<class "Configuration.lvclass">, "UI Cluster"=w418:T14)
            n144 = call <userlib>:"Write Configuration.vi"("error in (no error)"=w415, "Variant"=w418, "Configuration in"=w416) -> ("error out"=w417:errorcluster)  [unwired: 7 in, 1 out]
            n145 = call <vilib>:"Add State(s) to Queue__jki_lib_state_machine.vi"("State(s) in (\"\")"=w422) -> ("States Out"=w421:string)  [unwired: 14 in]
          }
          frame "Configuration: Read UI Config File" {
            # "Do not put any code in this frame.\n(It is a separator no-op. You can make a copy of this frame to create a new UI frame)"
            n146 = Unbundle By Name(w425) -> ("UI Cluster"=w428:T14, "Configuration"=w431:refnum<class "Configuration.lvclass">)
            n147 = call <userlib>:"Read Configuration.vi"("INI Fomatted Cluster Type"=w428, "error in (no error)"=w427, "Configuration in"=w431) -> ("error out"=w430:errorcluster, "Configuration"=w429:variant)  [unwired: 6 in, 1 out]
            n148 = Variant To Data(error in=w430, type=w428, Variant=w429) -> (data=w424:T14, error out=w426:errorcluster)
            n149 = Bundle By Name(cluster=w425, "UI Cluster"=w424) -> (w423:T16)
            n150 = call <vilib>:"Add State(s) to Queue__jki_lib_state_machine.vi"("State(s) in (\"\")"=w434) -> ("States Out"=w433:string)  [unwired: 14 in]
          }
          frame "---------- Action ----------" {
            n151 = Unbundle By Name(w436) -> ("Instrument"=w437:refnum<class "Inst.Krohn-Hite-7008.lvclass">)
            n152 = Bundle By Name(cluster=w436, "Instrument"=w437) -> (w435:T16)
            n153 = call <vilib>:"Add State(s) to Queue__jki_lib_state_machine.vi"("State(s) in (\"\")"=w441) -> ("States Out"=w440:string)  [unwired: 14 in]
          }
          frame "Action: Notify UI Closed" {
            # "Notify that the UI has been closed"
            n154 = Unbundle By Name(w442) -> ("Instrument UI"=w445:refnum<class "Inst UI.Krohn-Hite-7008.lvclass">)
            n155 = call <vilib>:"Hide.vi"("error in (no error)"=w444, "SMO.UI"=w445) -> ("error out"=w443:errorcluster)  [unwired: 8 in, 1 out]
            n156 = call <vilib>:"Add State(s) to Queue__jki_lib_state_machine.vi"("State(s) in (\"\")"=w448) -> ("States Out"=w447:string)  [unwired: 14 in]
          }
          frame "Action: getAll" {
            n157 = Unbundle By Name(w452) -> ("getAll"=w450:T13, "Instrument"=w455:refnum<class "Inst.Krohn-Hite-7008.lvclass">)
            n158 = call "GET ALL.vim"("type"=w450, "error in (no error)"=w453, "Instrument in"=w455) -> ("error out"=w457:errorcluster, "getAll"=w449:T13, "Instrument out"=w451:refnum<class "Inst.Krohn-Hite-7008.lvclass">)  [unwired: 6 in]
            n159 = Bundle By Name(cluster=w452, "Instrument"=w451, "getAll"=w449) -> (w454:T16)
            n160 = call <vilib>:"Add State(s) to Queue__jki_lib_state_machine.vi"("State(s) in Front (\"\")"="" ("State(s) in Front (\"\")"), "State(s) in (\"\")"=w460) -> ("States Out"=w459:string)  [unwired: 13 in]
          }
          frame "Action: Open" {
            n161 = Unbundle By Name(w467) -> ("Instrument"=w465:refnum<class "Inst.Krohn-Hite-7008.lvclass">)
            n162 = call <userlib>:"Write Client Type.vi"("error in (no error)"=w462, "Client Type"=Client_Type--Enum."Local", "Instrument in"=w465) -> ("error out"=w463:errorcluster, "Instrument out"=w464:refnum<class "Inst.Krohn-Hite-7008.lvclass">)  [unwired: 7 in]
            n163 = call-dynamic "Open.vi"("error in (no error)"=w463, "Inst.Krohn-Hite-7008 in"=w464) -> ("error out"=w470:errorcluster, "Inst.Krohn-Hite-7008 out"=w466:refnum<class "Inst.Krohn-Hite-7008.lvclass">)  [unwired: 8 in]
            n164 = Bundle By Name(cluster=w467, "Instrument"=w466) -> (w468:T16)
            n165 = call <vilib>:"Add State(s) to Queue__jki_lib_state_machine.vi"("State(s) in Front (\"\")"="" ("State(s) in Front (\"\")"), "State(s) in (\"\")"=w473) -> ("States Out"=w472:string)  [unwired: 13 in]
          }
          frame "Action: Close" {
            n166 = Unbundle By Name(w475) -> ("Instrument"=w478:refnum<class "Inst.Krohn-Hite-7008.lvclass">)
            n167 = call-dynamic "Close.vi"("error in (no error)"=w476, "Inst.Krohn-Hite-7008 in"=w478) -> ("error out"=w480:errorcluster, "Inst.Krohn-Hite-7008 out"=w474:refnum<class "Inst.Krohn-Hite-7008.lvclass">)  [unwired: 8 in]
            n168 = Bundle By Name(cluster=w475, "Instrument"=w474) -> (w477:T16)
            n169 = call <vilib>:"Add State(s) to Queue__jki_lib_state_machine.vi"("State(s) in Front (\"\")"="" ("State(s) in Front (\"\")"), "State(s) in (\"\")"=w483) -> ("States Out"=w482:string)  [unwired: 13 in]
          }
          frame "Action: Send Message to Instrument" {
            # "\"local\""
            # "Send a message (command, data, etc) to the Instrument:process.vi"
            n170 = Unbundle By Name(w488) -> ("Instrument"=w487:refnum<class "Inst.Krohn-Hite-7008.lvclass">)
            n171 = call <userlib>:"Instrument.MessageToProcess.vi"("error in (no error)"=w485, "Instrument"=w487) -> ("error out"=w484:errorcluster, "Instrument out"=w486:refnum<class "Inst.Krohn-Hite-7008.lvclass">)  [unwired: 8 in]
            n172 = Bundle By Name(cluster=w488, "Instrument"=w486) -> (w489:T16)
            n173 = call <vilib>:"Add State(s) to Queue__jki_lib_state_machine.vi"("State(s) in Front (\"\")"="" ("State(s) in Front (\"\")"), "State(s) in (\"\")"=w493) -> ("States Out"=w492:string)  [unwired: 13 in]
          }
          frame "Action: GetConfig" {
            # "\"local\""
            # "Send a message (command, data, etc) to the Instrument:process.vi"
            n174 = Unbundle By Name(w499) -> ("Instrument"=w498:refnum<class "Inst.Krohn-Hite-7008.lvclass">)  [unwired: 1 out]
            n175 = call <userlib>:"Instrument.MessageToProcess.vi"("error in (no error)"=w496, "Command"="GetConfig", "Instrument"=w498) -> ("error out"=w495:errorcluster, "Instrument out"=w497:refnum<class "Inst.Krohn-Hite-7008.lvclass">)  [unwired: 7 in]
            n176 = Bundle By Name(cluster=w499, "Instrument"=w497) -> (w500:T16)
            n177 = call <vilib>:"Add State(s) to Queue__jki_lib_state_machine.vi"("State(s) in Front (\"\")"="" ("State(s) in Front (\"\")"), "State(s) in (\"\")"=w504) -> ("States Out"=w503:string)  [unwired: 13 in]
          }
          frame "Action: Set Channel Data" {
            # "\"local\""
            # "Send a message (command, data, etc) to the Instrument:process.vi"
            n178 = Unbundle By Name(w511) -> ("Instrument"=w510:refnum<class "Inst.Krohn-Hite-7008.lvclass">)  [unwired: 1 out]
            n179 = call <userlib>:"Instrument.MessageToProcess.vi"("error in (no error)"=w508, "Data"="Channel Setting", "Command"="Set Channel Data", "Instrument"=w510) -> ("error out"=w507:errorcluster, "Instrument out"=w509:refnum<class "Inst.Krohn-Hite-7008.lvclass">)  [unwired: 6 in]
            n180 = Bundle By Name(cluster=w511, "Instrument"=w509) -> (w512:T16)
            n181 = call <vilib>:"Add State(s) to Queue__jki_lib_state_machine.vi"("State(s) in Front (\"\")"="" ("State(s) in Front (\"\")"), "State(s) in (\"\")"=w516) -> ("States Out"=w515:string)  [unwired: 13 in]
          }
          frame "Action: Send Message to Child" {
            # "Send a message (command, data, etc) to the Instrument.Child:process.vi"
            n182 = Unbundle By Name(w521) -> ("Instrument"=w520:refnum<class "Inst.Krohn-Hite-7008.lvclass">)  [unwired: 1 out]
            n183 = call "Inst.Krohn-Hite-7008.MessageToProcess.vi"("error in (no error)"=w518, "Inst.Krohn-Hite-7008 in"=w520) -> ("error out"=w517:errorcluster, "Inst.Krohn-Hite-7008 out"=w519:refnum<class "Inst.Krohn-Hite-7008.lvclass">)  [unwired: 8 in]
            n184 = Bundle By Name(cluster=w521, "Instrument"=w519) -> (w522:T16)
            n185 = call <vilib>:"Add State(s) to Queue__jki_lib_state_machine.vi"("State(s) in Front (\"\")"="" ("State(s) in Front (\"\")"), "State(s) in (\"\")"=w526) -> ("States Out"=w525:string)  [unwired: 13 in]
          }
        }
      }
    }
    frame Error {
    }
  }
  n186 = call-parent "Process.vi"("error in"=w5, "Instrument UI in"=w4) -> ("error out"=w2:errorcluster, "Instrument UI out"=→"Inst UI.Krohn-Hite-7008 out":refnum<class "Inst UI.Krohn-Hite-7008.lvclass">)  [unwired: 8 in]
  n187 = Merge Errors(w2, w1) -> (→"error out":errorcluster)
